vi "Write OCP_Mode.vi"(8 "error in":errorcluster, 10 "OCP Mode":T1, 11 "PowerSupply in":refnum<class "PowerSupply.lvclass">) -> (0 "error out":errorcluster, 3 "PowerSupply out":refnum<class "PowerSupply.lvclass">)   [LabVIEW 2019, in "PowerSupply.lvlib" / "PowerSupply.lvclass"]
uses:
  Library/PowerSupply.lvclass
  Custom Controls/OCP Mode.ctl
  Library/PowerSupply.lvclass/PowerSupply.ctl
  Read Settings.vi
  Write Settings.vi
  builds/Engine/Engine.lvlibp/Project/Engine.lvclass
  builds/Instruments/Instruments.lvlibp/Library/Instruments.lvclass
  builds/Instruments/Instruments.lvlibp/Private/Polymorphic/Special/Event from Enum.vi
  builds/Instruments/Instruments.lvlibp
  C:/Users/Public/Documents/Development/builds/Instruments/Instruments.lvlibp/Library/Instruments.lvclass
  C:/Users/Public/Documents/Development/builds/Tools/Config.lvlibp/Config.lvclass
  C:/Users/Public/Documents/Development/builds/Engine/Engine.lvlibp/Project/Engine.lvclass
  C:/Users/Public/Documents/Development/builds/Engine/Panel Manager.lvlibp/Panel Actor/Panel Actor.lvclass
  C:/Users/Public/Documents/Development/builds/Engine/Monitored Actor.lvlibp/Monitored Actor/Monitored Actor/Monitored Actor.lvclass
  C:/Users/Public/Documents/Development/builds/Engine/Actor Framework.lvlibp/1abvi3w/vi.lib/ActorFramework/Actor/Actor.lvclass
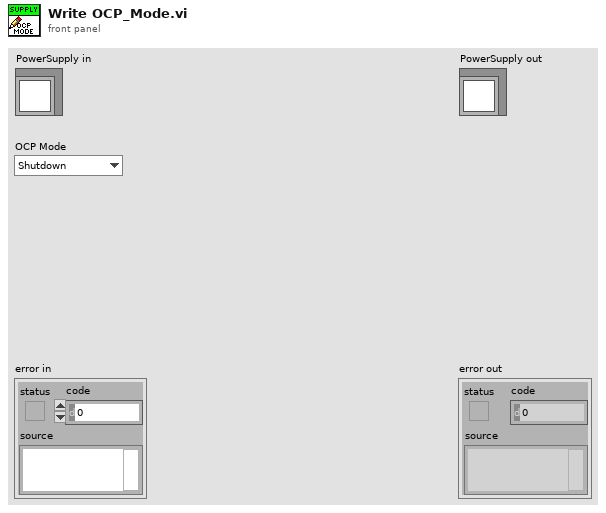
[diagram p1: front panel]
types:
  T1 = typedef "PowerSupply.lvlib/PowerSupply.lvclass/OCP Mode.ctl" = enum16{"Shutdown", "Foldback"}
  T2 = typedef "PowerSupply.lvlib/PowerSupply.lvclass/Settings.ctl" = cluster{"Voltage":dbl, "Current":dbl, "Output":bool, "OverVolt_Protect":dbl, "OverCurrent_Protect":dbl, "OVP":bool, "OCP":bool, "Interlock":bool, "Volt_Ramp":dbl, "Current_Ramp":dbl, "Sense Point":T3, "OCP Mode":T1}
  T3 = typedef "PowerSupply.lvlib/PowerSupply.lvclass/Sense Point.ctl" = enum16{"Local", "Remote"}
  T4 = cluster{"Timestamp":timestamp, "Description":string, "Data":string}
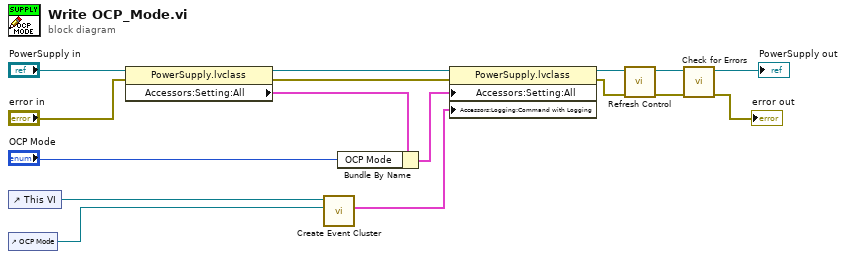
[diagram p0: block diagram]
diagram:
  n1 = control-ref of="This VI"() -> (w3:refnum<vi>)
  n2 = control-ref of="OCP Mode"() -> (w2:refnum<vi>)
  n3 = property class="PowerSupply.lvclass"(reference="PowerSupply in", error in="error in") -> (reference out=w9:refnum<class "PowerSupply.lvclass">, error out=w15:errorcluster, "Accessors:Setting:All"=w13:T2)
  n4 = call-poly "Create Event Cluster.vi"("Value"=w2, "VI Refnum"=w3) -> ("Event Data"=w1:T4)  [unwired: 9 in]
  n5 = Bundle By Name(cluster=w13, "OCP Mode"="OCP Mode") -> (w14:T2)
  n6 = property class="PowerSupply.lvclass"(reference=w9, error in=w15, "Accessors:Setting:All"=w14, "Accessors:Logging:Command with Logging"=w1) -> (reference out=w10:refnum<class "PowerSupply.lvclass">, error out=w16:errorcluster)
  n7 = call "Refresh Control.vi"("error in"=w16, "PowerSupply in"=w10) -> ("error out"=w11:errorcluster, "PowerSupply out"=w12:refnum<class "PowerSupply.lvclass">)  [unwired: 8 in]
  n8 = call "Check for Errors.vi"("error in"=w11, "Engine in"=w12) -> ("error out"=→"error out":errorcluster, "Engine out"=→"PowerSupply out":refnum<class "PowerSupply.lvclass">)  [unwired: 8 in]
